vi "Read Number of subscriptions.vi"(8 "error in (no error)":errorcluster, 11 "SubscriptionDetailsParent in":refnum<class "SubscriptionDetailsParent.lvclass">) -> (0 "error out":errorcluster, 2 "Number of subscriptions":u64, 3 "SubscriptionDetailsParent out":refnum<class "SubscriptionDetailsParent.lvclass">)   [LabVIEW 2020, in "wamplv.lvlib" / "SubscriptionDetailsParent.lvclass"]
uses:
  SubscriptionDetailsParent.lvclass
  SubscriptionDetailsParent.lvclass/SubscriptionDetailsParent.ctl
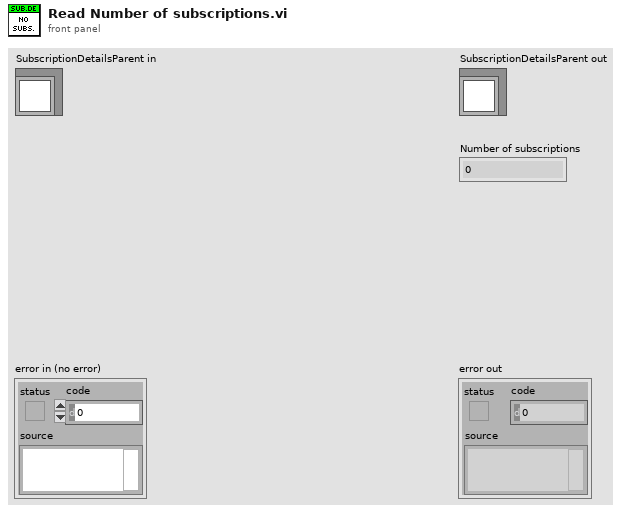
[diagram p1: front panel]
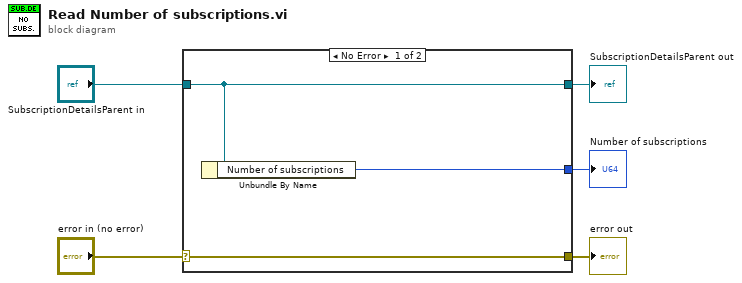
[diagram p0: block diagram]
diagram:
  n1 = case shown="No Error" "error in (no error)" {
    selector: "error in (no error)" -> [w8 w9]
    tunnel: [w8 w9] -> w4
    tunnel: [w7 w10] -> w2
    tunnel: "SubscriptionDetailsParent in" -> [w7 w10]
    tunnel: [w6 _] -> w1
    frame No Error {
      n2 = Unbundle By Name(w7) -> ("Number of subscriptions"=w6:u64)
    }
    frame Error {
    }
  }
  "error out" <- w4
  "SubscriptionDetailsParent out" <- w2
  "Number of subscriptions" <- w1
